vi "Implement Dynamic Dispatch VIs.vi"(8 "error in (no error)":errorcluster, 11 "Mock Class Generator In":refnum<class "Responsive Mock Class Generator.lvclass">) -> (0 "error out":errorcluster, 3 "Mock Class Generator Out":refnum<class "Responsive Mock Class Generator.lvclass">)   [LabVIEW 2020, in "Responsive Mock Class Generator.lvclass"]
uses:
  Responsive Mock Class Generator.lvclass
  Responsive Mock Class Generator.lvclass/Responsive Mock Class Generator.ctl
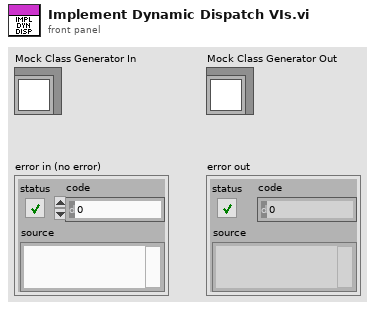
[diagram p1: front panel]
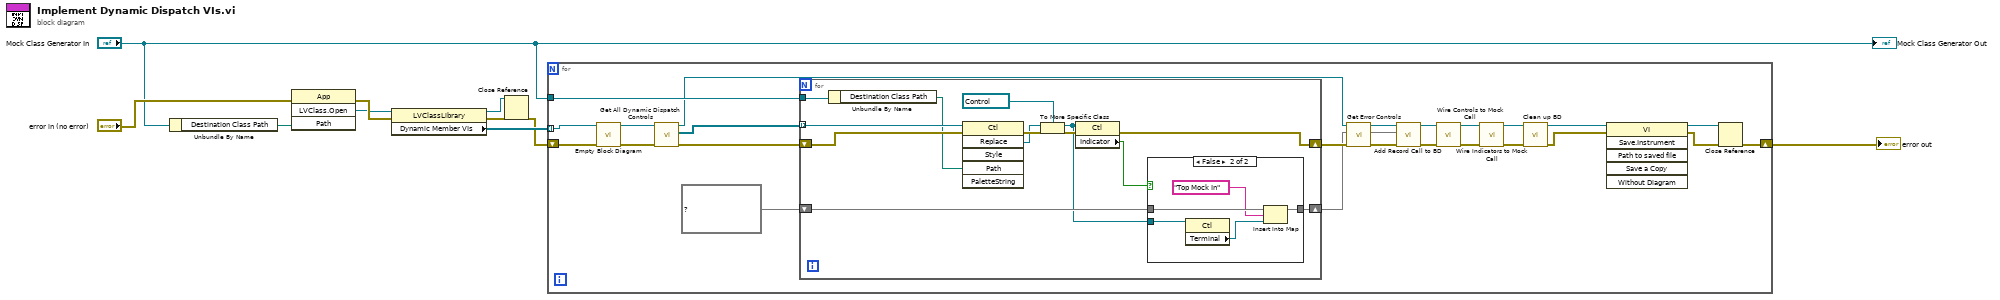
[diagram p0: block diagram]
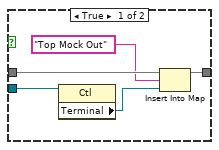
[diagram p2: hidden frame]
diagram:
  n1 = Unbundle By Name("Mock Class Generator In") -> ("Destination Class Path"=w10:path)
  n2 = invoke class="App" method="LVClass.Open"(error in="error in (no error)", "Path"=w10) -> (error out=w9:errorcluster, "LVClass.Open"=w4:refnum<vi>)  [unwired: 2 in, 2 out]
  n3 = property class="LVClassLibrary"(reference=w4, error in=w9) -> (reference out=w5:refnum<vi>, error out=w6:errorcluster, "Dynamic Member VIs"=w7:refnum<vi>[])
  n4 = Close Reference(reference=w5, error in (no error)=w6) -> (error out=w3:errorcluster)
  n5 = for {
    tunnel: w7 -> [w21] mode=indexing
    tunnel: "Mock Class Generator In" -> [w34]
    shift-right: [w32] -> w1
    shift-left: w3 -> [w17]
    n6 = call "Empty Block Diagram.vi"("error in (no error)"=w17, "VI in"=w21) -> ("error out"=w18:errorcluster, "reference out"=w31:refnum<vi>)  [unwired: 8 in]
    n7 = call "Get All Dynamic Dispatch Controls.vi"("error in (no error)"=w18, "VI in"=w31) -> ("error out"=w35:errorcluster, "Dynamic Dispatch Controls"=w33:refnum<vi>[], "reference out"=w29:refnum<vi>)  [unwired: 7 in]
    n8 = for {
      tunnel: w33 -> [w48] mode=indexing
      shift-right: [w40] -> w30
      shift-left: w35 -> [w47]
      tunnel: w34 -> [w46]
      shift-right: [w38] -> w25
      shift-left: map{string, refnum<vi>} {} ("map") -> [w39]
      n9 = Unbundle By Name(w46) -> ("Destination Class Path"=w45:path)
      n10 = invoke class="Ctl" method="Replace"(reference=w48, error in=w47, "Path"=w45) -> (error out=w44:errorcluster, "Replace"=w42:refnum<vi>)  [unwired: 3 in, 4 out]
      n11 = To More Specific Class(target class=refnum<vi> refnum ("reference out"), reference=w42, error in=w44) -> (specific class reference=w36:refnum<vi>, error out=w43:errorcluster)
      n12 = property class="Ctl"(reference=w36, error in=w43) -> (error out=w40:errorcluster, "Indicator"=w37:bool)  [unwired: 1 out]
      n13 = case shown="False" w37 {
        tunnel: w39 -> [w53 w58]
        tunnel: [w52 w57] -> w38
        tunnel: w36 -> [w50 w55]
        frame True {
          n14 = property class="Ctl"(reference=w50) -> ("Terminal"=w49:refnum<vi>)  [unwired: 1 in, 2 out]
          n15 = Insert Into Map(map in=w53, key="Top Mock Out", value=w49) -> (map out=w52:map{string, refnum<vi>})  [unwired: 2 out]
        }
        frame False {
          n16 = property class="Ctl"(reference=w55) -> ("Terminal"=w54:refnum<vi>)  [unwired: 1 in, 2 out]
          n17 = Insert Into Map(map in=w58, key="Top Mock In", value=w54) -> (map out=w57:map{string, refnum<vi>})  [unwired: 2 out]
        }
      }
    }
    n18 = call "Get Error Controls.vi"("error in (no error)"=w30, "map"=w25, "VI in"=w29) -> ("error out"=w27:errorcluster, "map out"=w24:map{string, refnum<vi>}, "reference out"=w28:refnum<vi>)  [unwired: 6 in]
    n19 = call "Add Record Call to BD.vi"("error in (no error)"=w27, "map"=w24, "VI in"=w28) -> ("error out"=w19:errorcluster, "VI out"=w14:refnum<vi>)  [unwired: 7 in]
    n20 = call "Wire Controls to Mock Call.vi"("error in (no error)"=w19, "VI in"=w14) -> ("error out"=w15:errorcluster, "VI out"=w12:refnum<vi>)  [unwired: 8 in]
    n21 = call "Wire Indicators to Mock Call.vi"("error in (no error)"=w15, "VI in"=w12) -> ("error out"=w13:errorcluster, "VI out"=w11:refnum<vi>)  [unwired: 8 in]
    n22 = call "Clean up BD.vi"("error in (no error)"=w13, "VI in"=w11) -> ("error out"=w20:errorcluster, "VI out"=w23:refnum<vi>)  [unwired: 8 in]
    n23 = invoke class="VI" method="Save.Instrument"(reference=w23, error in=w20) -> (reference out=w22:refnum<vi>, error out=w16:errorcluster)  [unwired: 4 in, 4 out]
    n24 = Close Reference(reference=w22, error in (no error)=w16) -> (error out=w32:errorcluster)
  }
  "error out" <- w1
  "Mock Class Generator Out" <- "Mock Class Generator In"
